vi "USRP RX.vi"() -> ()   [LabVIEW 2022 SP3]
uses:
  <instrlib>/niUSRP/niUSRP Fetch Rx Data (CDB Cluster).vi
  <vilib>/addons/Modulation/niAMT.lvlib
panel:
  out "real Waveform":cluster{"t0":dbl, "dt":dbl, "Y":dbl[]}(graph)
  out "imaginary Waveform":cluster{"t0":dbl, "dt":dbl, "Y":dbl[]}(graph)
  in  "number of samples":i64
  out "coerced gain":dbl format="%#_6f"
  out "coerced carrier frequency":dbl=100000.0 format="%#_6p"
  out "coerced IQ rate":dbl=100000.0 format="%#_6p"
  in  "active antenna":string
  in  "gain":dbl format="%#_6f"
  in  "carrier frequency":dbl=100000.0 format="%#_6p"
  in  "IQ rate":dbl=100000.0 format="%#_6p"
  out "error out":errorcluster
  in  "device names":refnum<k15>
  in  "stop":bool
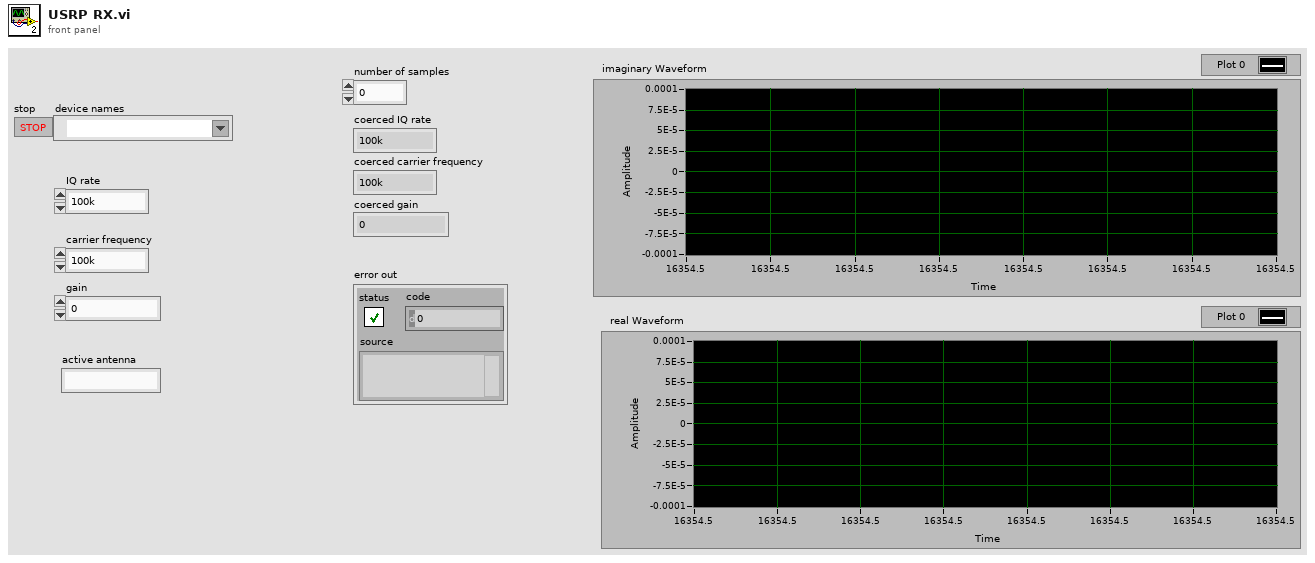
[diagram p1: front panel]
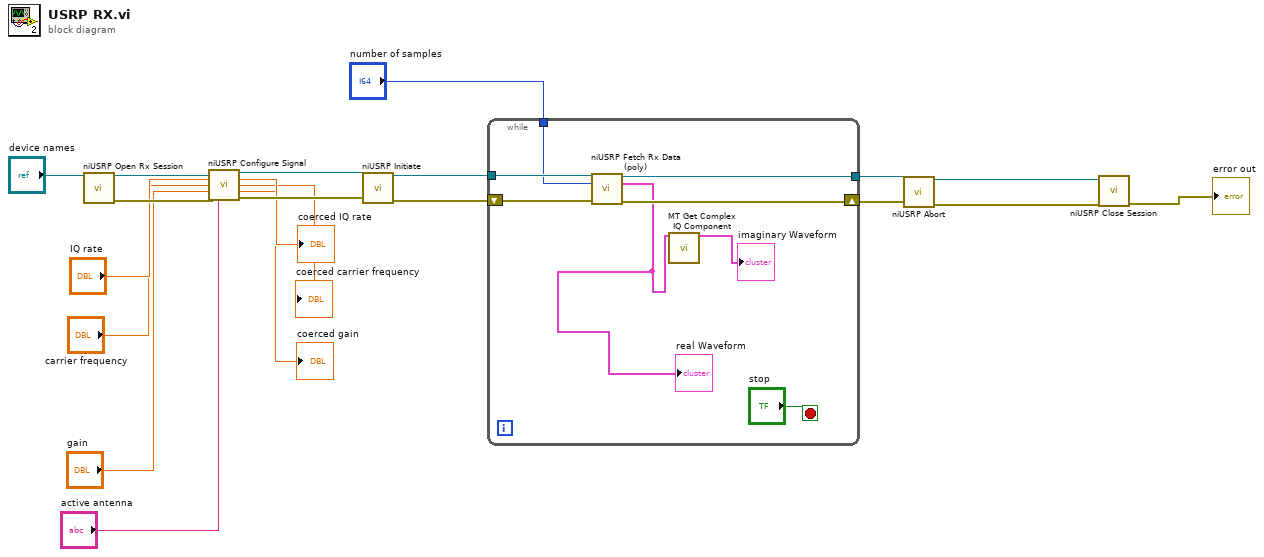
[diagram p0: block diagram]
diagram:
  n1 = call <instrlib>:"niUSRP Open Rx Session.vi"("device names"="device names") -> ("session handle out"=w19:refnum<k15>, "error out"=w14:errorcluster)  [unwired: 13 in]
  n2 = call <instrlib>:"niUSRP Configure Signal.vi"("session handle"=w19, "IQ rate"="IQ rate", "carrier frequency"="carrier frequency", "gain"="gain", "error in (no error)"=w14, "active antenna"="active antenna") -> ("session handle out"=w18:refnum<k15>, "coerced IQ rate"=→"coerced IQ rate":dbl, "coerced carrier frequency"=→"coerced carrier frequency":dbl, "coerced gain"=→"coerced gain":dbl, "error out"=w13:errorcluster)  [unwired: 5 in]
  n3 = call <instrlib>:"niUSRP Initiate.vi"("session handle"=w18, "error in (no error)"=w13) -> ("session handle out"=w17:refnum<k15>, "error out"=w12:errorcluster)  [unwired: 12 in]
  n4 = while {
    tunnel: w17 -> [w27]
    tunnel: [w26] -> w16
    shift-right: [w24] -> w11
    shift-left: w12 -> [w25]
    tunnel: "number of samples" -> [w23]
    stop <- "stop" stop-if-true
    n5 = call-poly <instrlib>:"niUSRP Fetch Rx Data (poly).vi"("session handle"=w27, "number of samples"=w23, "error in (no error)"=w25) -> ("session handle out"=w26:refnum<k15>, "data"=w21:cluster{"t0":dbl, "dt":dbl, "Y":cdb[]}, "error out"=w24:errorcluster)  [unwired: 9 in, 1 out]
    "real Waveform" <- w21
    n6 = call <vilib>:"MT Get Complex IQ Component.vi"("IQ data (complex) in"=w21) -> ("IQ data (complex) out"=→"imaginary Waveform":cluster{"t0":dbl, "dt":dbl, "Y":cdb[]})  [unwired: 12 in, 2 out]
  }
  n7 = call <instrlib>:"niUSRP Abort.vi"("session handle"=w16, "error in (no error)"=w11) -> ("session handle out"=w15:refnum<k15>, "error out"=w10:errorcluster)  [unwired: 12 in]
  n8 = call <instrlib>:"niUSRP Close Session.vi"("session handle"=w15, "error in (no error)"=w10) -> ("error out"=→"error out":errorcluster)  [unwired: 13 in]
